vi "IMAQ Mask.vi"() -> ()   [LabVIEW 2012, in "LightPipes.lvlib"]
uses:
  LightPipes.lvlib
  <vilib>/vision/NI_Vision_Development_Module.lvlib
panel:
  in  "Image Type":T1 items=["Grayscale (U8)", "Grayscale (I16)", "Grayscale (SGL)", "Complex (CSG)", "RGB (U32)", "HSL (U32)", "RGB (U64)", "Grayscale (U16)"]
  out "Noise Value":i32=1
  in  "Noise Remove":bool
  in  "Save":bool
  in  "Input Image Path":path=path "C:/Users/Tri/Documents/Lightpipes/LabView/beam images/OSP Midfield.png"
  out "Image":T2(plugin-control)
  in  "Stop":bool
  in  "Mask":bool
  out "Mask":T2(plugin-control)
  # "1. Select the Image File\n2. Select the Region of Interest (ROI)\n3. Press Mask\n4. Press Save to save the masked picture\n5. Press Return to exit"
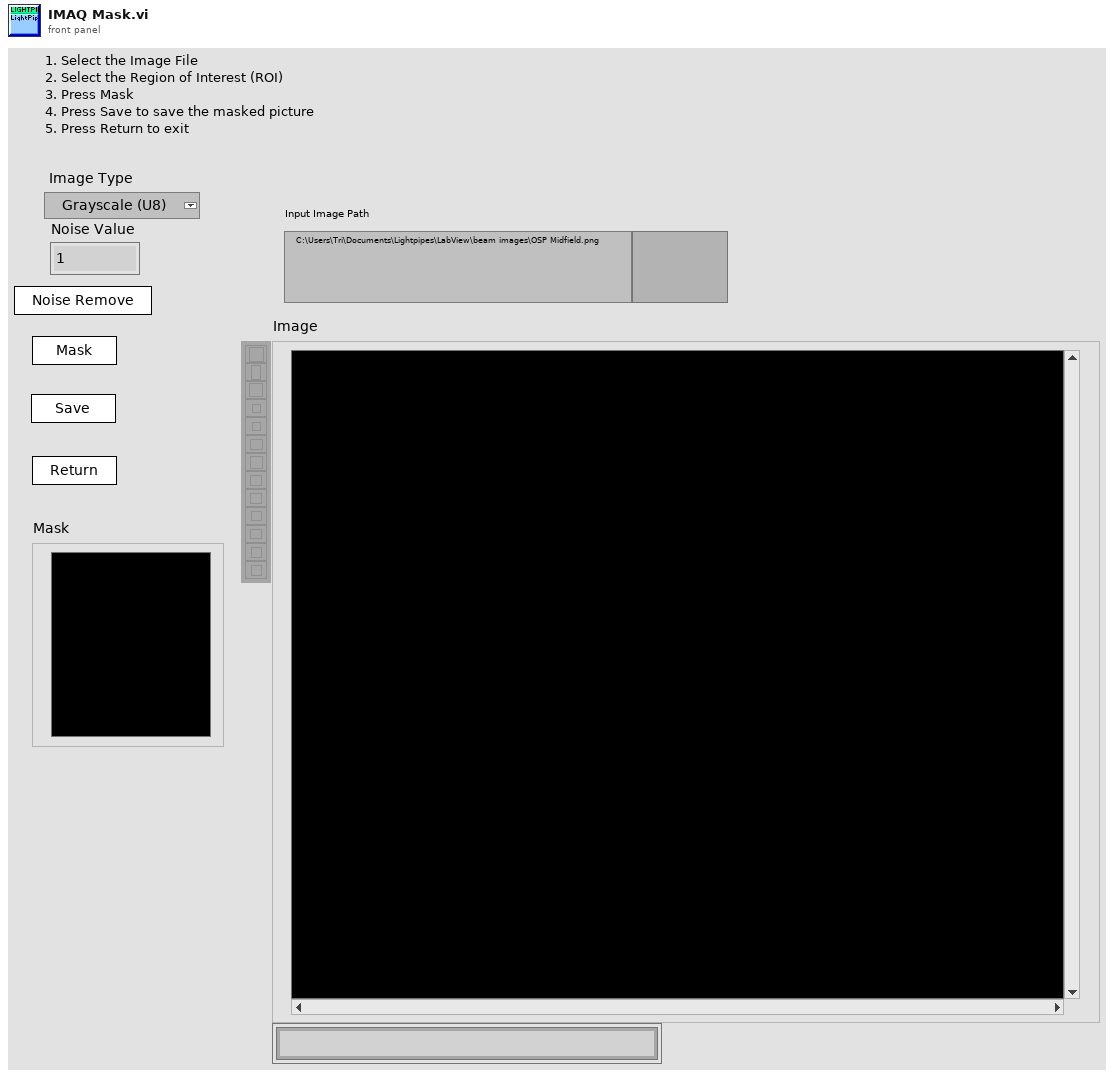
[diagram p1: front panel]
types:
  T1 = typedef "Image Type" = u32
  T2 = typedef "IMAQ Image.ctl" = refnum<image>
  T3 = cluster{"Global Rectangle":i32[], "Contours":cluster{"Contour Type":u32, "ROI Type":u32, "Points":i32[]}[]}
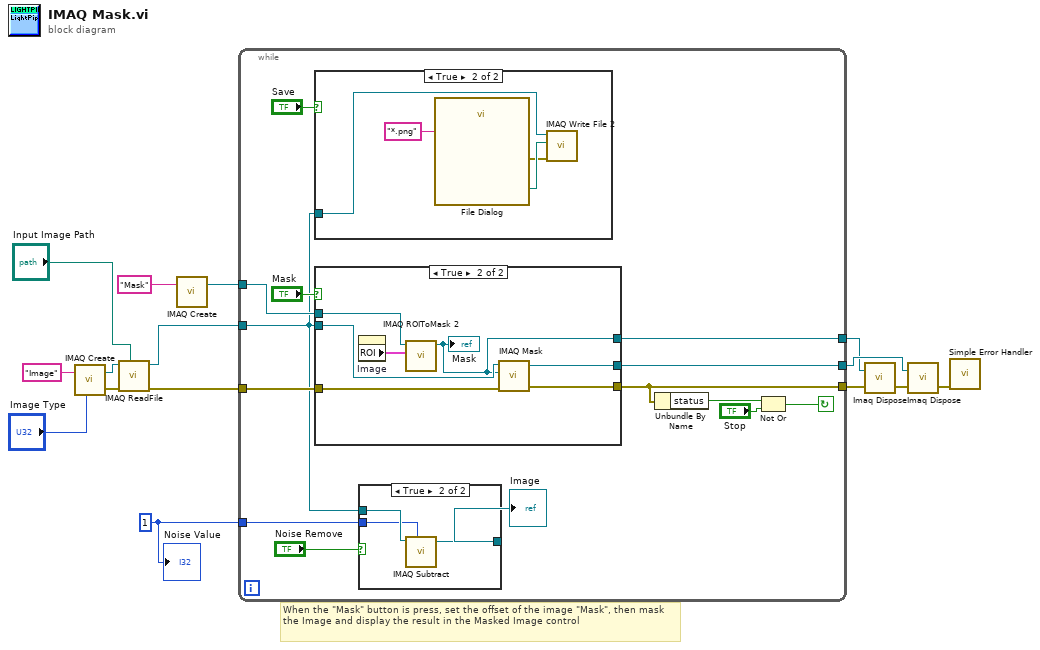
[diagram p0: block diagram]
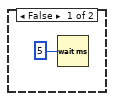
[diagram p3: hidden frame]
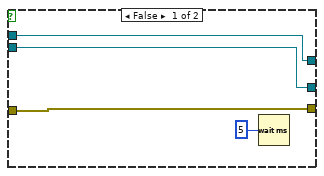
[diagram p4: hidden frame]
diagram:
  w2 = 1 ("Noise Value")
  # "When the \"Mask\" button is press, set the offset of the image \"Mask\", then mask the Image and display the result in the Masked Image control"
  n1 = call "IMAQ Create"("Image Name"="Image", "Image Type"="Image Type") -> ("New Image"=w9:T2, "error out"=w14:errorcluster)  [unwired: 2 in, 1 out]
  n2 = call "IMAQ ReadFile"("File Path"="Input Image Path", "error in (no error)"=w14, "Image"=w9) -> ("error out"=w13:errorcluster, "Image Out"=w3:T2)  [unwired: 2 in, 5 out]
  n3 = call "IMAQ Create"("Image Name"="Mask") -> ("New Image"=w10:T2)  [unwired: 3 in, 2 out]
  n4 = while {
    tunnel: w3 -> [w18]
    tunnel: w13 -> [w28]
    tunnel: [w27] -> w4
    tunnel: [w21] -> w8
    tunnel: [w23] -> w6
    tunnel: w10 -> [w19]
    tunnel: w2 -> [w17]
    stop <- w24 continue-if-true
    n5 = case shown="True" "Save" {
      tunnel: w18 -> [_ w36]
      frame False {
        n6 = Wait (ms)(milliseconds to wait=u32 5) -> ()  [unwired: 1 out]
      }
      frame True {
        n7 = call "File Dialog"("pattern (all files)"="*.png") -> ("selected path"=w38:path, "error out"=w35:errorcluster)  [unwired: 11 in, 2 out]
        n8 = call-poly "IMAQ Write File 2"("error in (no error)"=w35, "File Path"=w38, "Image"=w36) -> ()  [unwired: 7 in, 2 out]
      }
    }
    n9 = case shown="True" "Mask" {
      tunnel: w18 -> [w42 w49]
      tunnel: w28 -> [w41 w45]
      tunnel: [w42 w43] -> w21
      tunnel: [w41 w48] -> w27
      tunnel: [w39 w46] -> w23
      tunnel: w19 -> [w39 w44]
      frame False {
        n10 = Wait (ms)(milliseconds to wait=u32 5) -> ()  [unwired: 1 out]
      }
      frame True {
        n11 = property on="Image" class="ImageControl"() -> ("ROI"=w47:T3)  [unwired: 2 in, 2 out]
        n12 = call "IMAQ ROIToMask 2"("ROI Descriptor"=w47, "Image"=w44) -> ("Image Out"=w46:T2)  [unwired: 7 in, 2 out]
        "Mask" <- w46
        n13 = call "IMAQ Mask"("error in (no error)"=w45, "Image Mask"=w46, "Image Src"=w49) -> ("error out"=w48:errorcluster, "Image Dst Out"=w43:T2)  [unwired: 1 in, 1 out]
      }
    }
    n14 = case shown="True" "Noise Remove" {
      tunnel: w18 -> [w30 w33]
      tunnel: w17 -> [_ w32]
      tunnel: [w30 w31] -> w16
      frame False {
      }
      frame True {
        n15 = call "IMAQ Subtract"("Image Src A"=w33, "Constant"=w32) -> ("Image Dst Out"=w31:T2)  [unwired: 5 in, 1 out]
      }
    }
    "Image" <- w16
    n16 = Unbundle By Name(w27) -> ("status"=w26:bool)
    n17 = Not Or(1:"Stop", 2:w26) -> (0:w24:bool)
  }
  n18 = call "Imaq Dispose"("Image"=w6, "error in (no error)"=w4) -> ("error out"=w5:errorcluster)  [unwired: 1 in, 3 out]
  n19 = call "Imaq Dispose"("Image"=w8, "error in (no error)"=w5) -> ("error out"=w7:errorcluster)  [unwired: 1 in, 3 out]
  n20 = call <vilib>:"Simple Error Handler.vi"("error in (no error)"=w7) -> ()  [unwired: 1 in, 8 out]
  "Noise Value" <- w2
